vi "IMAQ FPGA Image Transfer to Target U64.vi"(7 "Write Timeout (ms)":i32=5000, 8 "error in (no error)":errorcluster, 9 "DMA FIFO Reference In":refnum<k20>, 10 "Maximum Pixels per Write":i32=-1, 11 "Image":T1) -> (0 "error out":errorcluster, 1 "DMA FIFO Reference Out":refnum<k20>, 3 "Image Out":T1)   [LabVIEW 2017, in "NI_VDM_FPGA_Basics.lvlib"]
doc: "Transfers an image from the host processor to the target FPGA via a DMA FIFO."
uses:
  <vilib>/visionFPGA/NI_VDM_FPGA_Basics.lvlib
  <vilib>/vision/Image Controls.llb/IMAQ Image.ctl
  <vilib>/rvi/errors/niLvFpgaAdjustHostInterfaceError.vi
  <vilib>/rvi/interface/nirviMethod/nirviMethod.xnode
  <vilib>/rvi/errors/niLvFpgaMergeErrorWithErrorCode.vi
  <vilib>/FPGAPlugInAG/Dynamic/niLvFpga_WriteFifo_Dynamic.vi
  <vilib>/FPGAPlugInAG/Dynamic/niLvFpga_AcquireWriteRegionFifo_Dynamic.vi
  <vilib>/vision/EDVR.llb/IMAQ ImageToEDVR 2D U64.vi
  nivissvc.dll
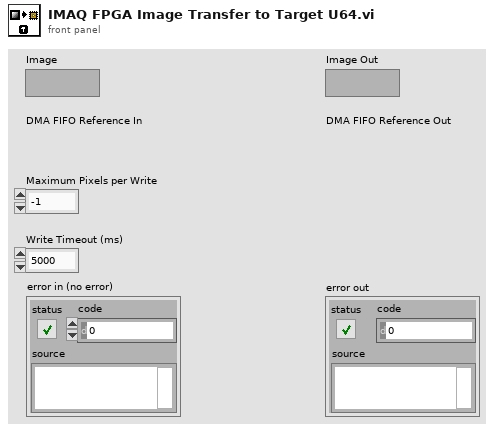
[diagram p1: front panel]
types:
  T1 = typedef "IMAQ Image.ctl" = refnum<image>
  T2 = typedef "Image Type" = u32
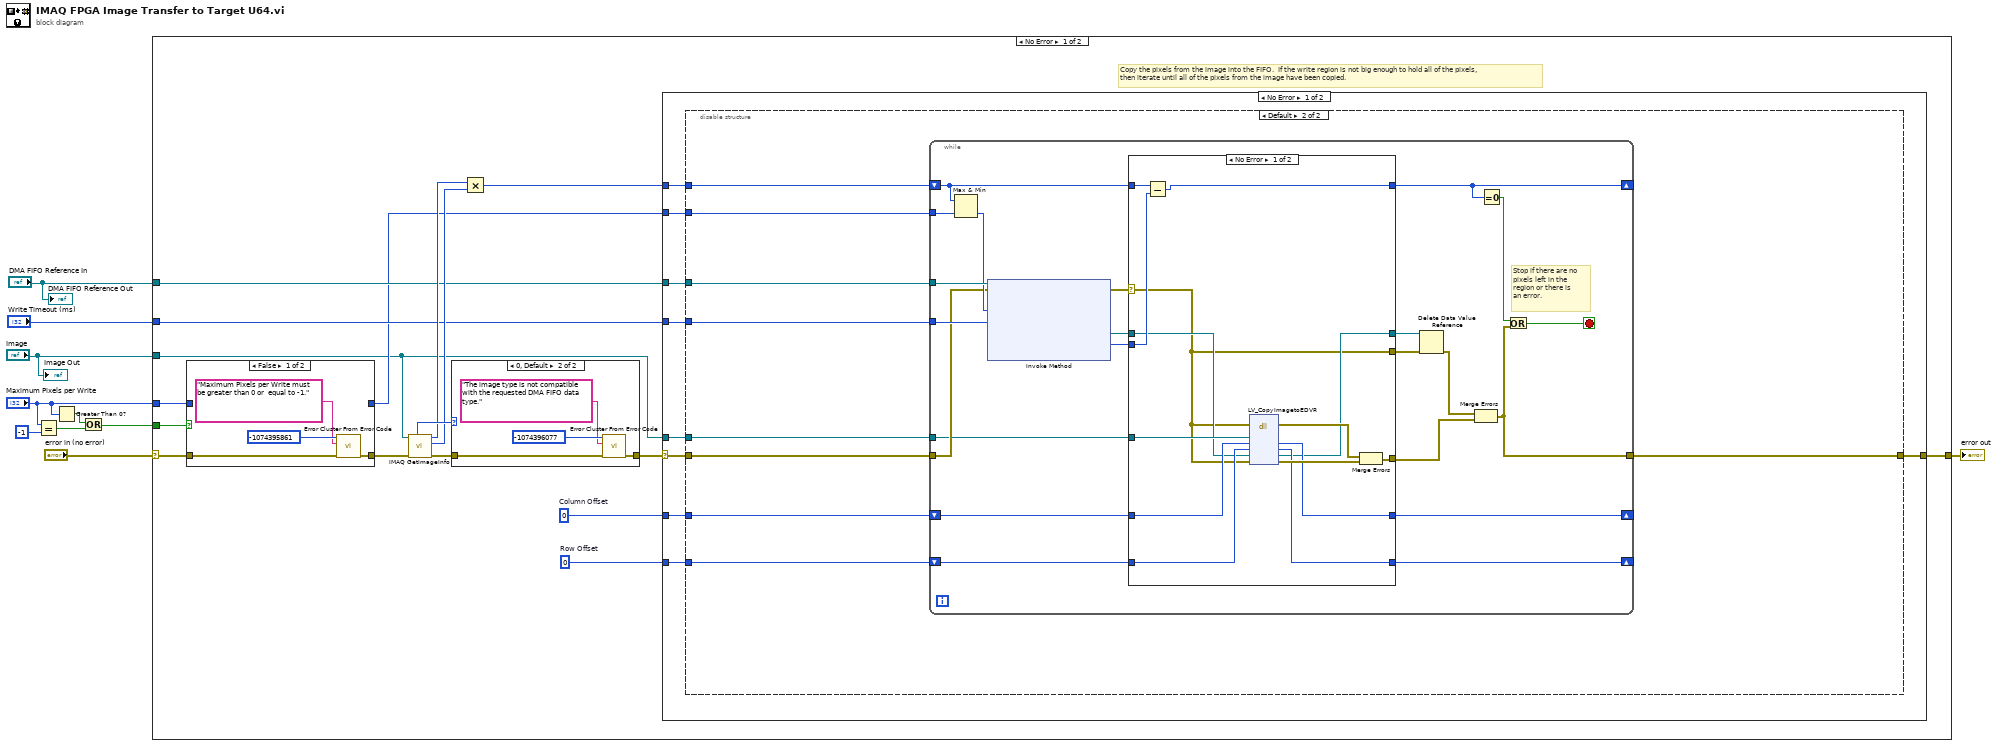
[diagram p0: block diagram]
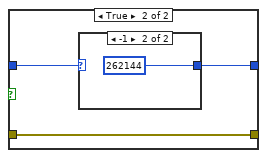
[diagram p2: hidden frame]
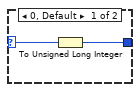
[diagram p3: hidden frame]
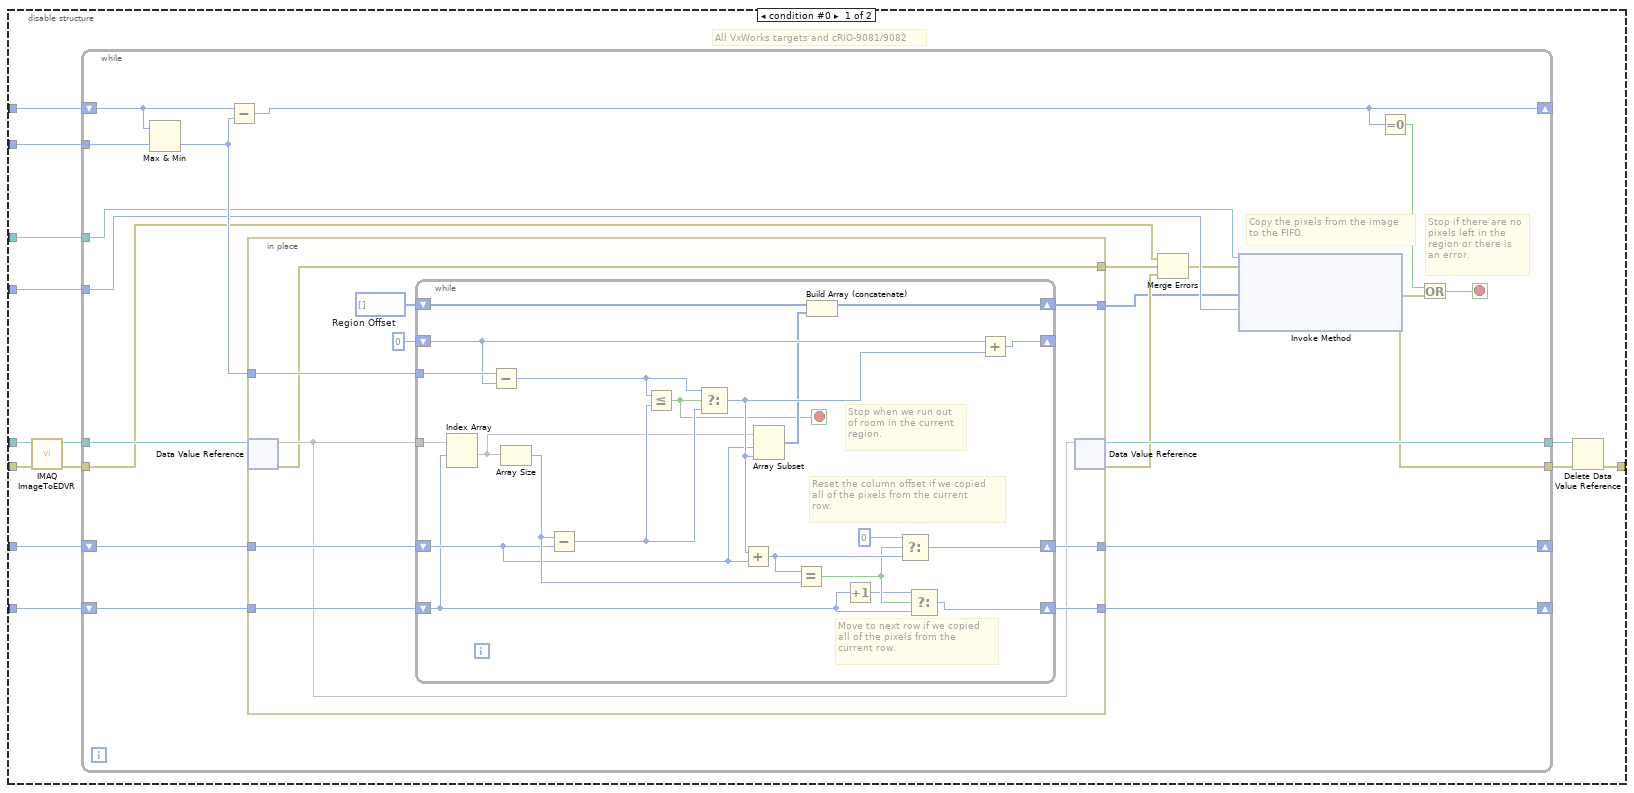
[diagram p4: hidden frame]
diagram:
  n1 = Equal?(x="Maximum Pixels per Write", y=-1) -> (x = y?=w6:bool)
  n2 = Greater Than 0?(x="Maximum Pixels per Write") -> (x > 0?=w7:bool)
  n3 = Or(x=w7, y=w6) -> (x .or. y?=w5:bool)
  n4 = case shown="No Error" "error in (no error)" {
    selector: "error in (no error)" -> [w11 w167]
    tunnel: "DMA FIFO Reference In" -> [w22 _]
    tunnel: "Write Timeout (ms)" -> [w21 _]
    tunnel: w5 -> [w18 _]
    tunnel: "Maximum Pixels per Write" -> [w15 _]
    tunnel: "Image" -> [w13 _]
    tunnel: [w12 w167] -> w2
    frame No Error {
      w19 = u32 0  # Row Offset
      w20 = u32 0  # Column Offset
      # "Copy the pixels from the image into the FIFO.  If the write region is not big enough to hold all of the pixels,\nthen iterate until all of the pixels from the image have been copied."
      n5 = case shown="False" w18 {
        tunnel: w11 -> [w29 w34]
        tunnel: [w28 w34] -> w17
        tunnel: w15 -> [_ w33]
        tunnel: [_ w32] -> w16
        frame False {
          n6 = call <vilib>:"Error Cluster From Error Code.vi"("error in (no error)"=w29, "error message (\"\")"="Maximum Pixels per Write must be greater than 0 or  equal to -1." ("error message (\"\")"), "error code (0)"=-1074395861) -> ("error out"=w28:errorcluster)  [unwired: 6 in]
        }
        frame True {
          n7 = case shown="-1" w33 {
            selector: w33 -> [w36 _]
            tunnel: [w35 u32 262144 ("Maximum Pixels per Write")] -> w32
            frame 0, Default {
              n8 = To Unsigned Long Integer(number=w36) -> (unsigned 32bit integer=w35:u32)
            }
            frame -1 {
            }
          }
        }
      }
      n9 = call "IMAQ GetImageInfo"("error in (no error)"=w17, "Image"=w13) -> ("error out"=w26:errorcluster, "Y Resolution"=w24:i32, "X Resolution"=w25:i32, "Image Type"=w27:T2)  [unwired: 2 in, 4 out]
      n10 = case shown="0, Default" w27 {
        tunnel: w26 -> [w162 w164]
        tunnel: [w162 w163] -> w14
        frame 6 {
          # "Allowed types are:\nRGB (U64)"
        }
        frame 0, Default {
          n11 = call <vilib>:"Error Cluster From Error Code.vi"("error in (no error)"=w164, "error message (\"\")"="The image type is not compatible with the requested DMA FIFO data type." ("error message (\"\")"), "error code (0)"=-1074396077) -> ("error out"=w163:errorcluster)  [unwired: 6 in]
        }
      }
      n12 = Multiply(x=w25, y=w24) -> (x*y=w23:i32)
      n13 = case shown="No Error" w14 {
        selector: w14 -> [w44 w161]
        tunnel: w23 -> [w39 _]
        tunnel: w20 -> [w45 _]
        tunnel: w19 -> [w46 _]
        tunnel: w22 -> [w41 _]
        tunnel: [w38 w161] -> w12
        tunnel: w16 -> [w40 _]
        tunnel: w21 -> [w42 _]
        tunnel: w13 -> [w43 _]
        frame No Error {
          n14 = disable-structure shown="Default" {
            disable-tunnel: w39 -> [w59 w119]
            disable-tunnel: w45 -> [w58 w118]
            disable-tunnel: w46 -> [w57 w117]
            disable-tunnel: w41 -> [w56 w116]
            disable-tunnel: [w47 w115] -> w38
            disable-tunnel: w40 -> [w55 w114]
            disable-tunnel: w42 -> [w54 w113]
            disable-tunnel: w44 -> [w52 w112]
            disable-tunnel: w43 -> [w53 w111]
            frame condition #0 {
              # "All VxWorks targets and cRIO-9081/9082"
              n15 = call-poly <vilib>:"IMAQ ImageToEDVR.vi"("error in (no error)"=w52, "Image"=w53) -> ("error out"=w50:errorcluster, "EDVR 2D U64"=w51:refnum<data-value>)  [unwired: 7 in, 1 out]
              n16 = while {
                shift-right: [w73] -> _
                shift-left: w59 -> [w70]
                tunnel: w51 -> [w79]
                shift-right: [w75] -> _
                shift-left: w58 -> [w77]
                shift-right: [w78] -> _
                shift-left: w57 -> [w76]
                tunnel: w56 -> [w64]
                tunnel: [w74] -> w49
                tunnel: [w62] -> w48
                tunnel: w55 -> [w69]
                tunnel: w54 -> [w65]
                tunnel: w50 -> [w60]
                stop <- w72 stop-if-true
                # "Copy the pixels from the image\nto the FIFO."
                # "Stop if there are no\npixels left in the \nregion or there is\nan error."
                n17 = Max & Min(x=w70, y=w69) -> (min(x,y)=w68:u32)  [unwired: 1 out]
                n18 = Subtract(x=w70, y=w68) -> (x-y=w73:u32)
                n19 = in-place {
                  in-place-border: w68 -> [w87]
                  in-place-border: [w89] -> w78
                  in-place-border: w77 -> [w86]
                  in-place-border: w76 -> [w84]
                  in-place-border: [w85] -> w75
                  in-place-border: [w81] -> w67
                  in-place-border: [w80] -> w61
                  w88 = u32 0  # Region Offset
                  n20 = in-place-dvr #1(w79) -> (w83:u64[][], w81:errorcluster)
                  n21 = while {
                    tunnel: w83 -> [w96]
                    shift-right: [w108] -> _
                    shift-left: w88 -> [w107]
                    tunnel: w87 -> [w110]
                    shift-right: [w101] -> w85
                    shift-left: w86 -> [w97]
                    shift-right: [w91] -> w80
                    shift-left: u8[] [] -> [w93]
                    shift-right: [w98] -> w89
                    shift-left: w84 -> [w94]
                    stop <- w90 stop-if-true
                    # "Stop when we run out\nof room in the current\nregion."
                    # "Reset the column offset if we copied\nall of the pixels from the current\nrow."
                    # "Move to next row if we copied\nall of the pixels from the\ncurrent row."
                    n22 = Index Array(array=w96, index (row)=w94) -> (element=w95:u64[])  [unwired: 1 in]
                    n23 = Subtract(x=w110, y=w107) -> (x-y=w109:u32)
                    n24 = Array Size(array=w95) -> (size(s)=w106:i32)
                    n25 = Subtract(x=w106, y=w97) -> (x-y=w104:u32)
                    n26 = Less Or Equal?(x=w109, y=w104) -> (x <= y?=w90:bool)
                    n27 = Select(t=w109, s=w90, f=w104) -> (s? t:f=w105:u32)
                    n28 = Add(x=w105, y=w97) -> (x+y=w102:u32)
                    n29 = Array Subset(array=w95, index=w97, length=w105) -> (w92:u64[])
                    n30 = Equal?(x=w102, y=w106) -> (x = y?=w100:bool)
                    n31 = Build Array (concatenate)(w93, w92) -> (w91:u64[])
                    n32 = Increment(x=w94) -> (x+1=w99:u32)
                    n33 = Select(t=u32 0 ("Elements In Region"), s=w100, f=w102) -> (s? t:f=w101:u32)
                    n34 = Select(t=w99, s=w100, f=w94) -> (s? t:f=w98:u32)
                    n35 = Add(x=w107, y=w105) -> (x+y=w108:u32)
                  }
                  n36 = in-place-dvr #1(w83) -> (w74:refnum<data-value>, w66:errorcluster)
                }
                n37 = Merge Errors(w60, w67, w66) -> (w63:errorcluster)
                n38 = xnode "Invoke Method"("FPGA VI Reference In"=w64, "error in"=w63, "Data"=w61, "Timeout (ms)"=w65) -> ("error out"=w62:errorcluster)  [unwired: 2 out]
                n39 = Equal To 0?(x=w73) -> (x = 0?=w71:bool)
                n40 = Or(x=w71, y=w62) -> (x .or. y?=w72:bool)
              }
              n41 = Delete Data Value Reference(data value reference=w49, error in=w48) -> (error out=w47:errorcluster)  [unwired: 1 out]
            }
            frame condition #1 (active) {
              n42 = while {
                shift-right: [w129] -> _
                shift-left: w119 -> [w124]
                shift-right: [w136] -> _
                shift-left: w118 -> [w138]
                shift-right: [w139] -> _
                shift-left: w117 -> [w137]
                tunnel: w116 -> [w135]
                tunnel: [w127] -> w115
                tunnel: w114 -> [w123]
                tunnel: w113 -> [w122]
                tunnel: w112 -> [w121]
                tunnel: w111 -> [w120]
                stop <- w128 stop-if-true
                # "Stop if there are no\npixels left in the \nregion or there is\nan error."
                n43 = Max & Min(x=w124, y=w123) -> (min(x,y)=w125:u32)  [unwired: 1 out]
                n44 = xnode "Invoke Method"("FPGA VI Reference In"=w135, "error in"=w121, "Number of Elements"=w125, "Timeout (ms)"=w122) -> ("error out"=w134:errorcluster, "Write Region Reference"=w141:refnum<data-value>, "Elements In Region"=w140:u32)  [unwired: 2 out]
                n45 = case shown="No Error" w134 {
                  selector: w134 -> [w142 w157]
                  tunnel: w124 -> [w155 w160]
                  tunnel: [w154 w160] -> w129
                  tunnel: w141 -> [w148 w156]
                  tunnel: w140 -> [w153 _]
                  tunnel: [w144 w158] -> w139
                  tunnel: w138 -> [w151 w159]
                  tunnel: w137 -> [w150 w158]
                  tunnel: [w145 w159] -> w136
                  tunnel: [w143 w156] -> w133
                  tunnel: [w142 w157] -> w132
                  tunnel: [w146 _] -> w130
                  tunnel: w120 -> [w152 _]
                  frame No Error {
                    n46 = Subtract(x=w155, y=w153) -> (x-y=w154:u32)
                    n47 = dll-call lib="nivissvc.*" fn="LV_CopyImagetoEDVR" label="LV_CopyImageToEDVR"(error in=w142, "image"=w152, "xImageOffset"=w151, "yImageOffset"=w150, "EDVR"=w148, "error"=w142) -> (error out=w149:errorcluster, "xImageOffset"=w145:u32, "yImageOffset"=w144:u32, "EDVR"=w143:refnum<data-value>, "error"=w147:errorcluster)  [unwired: 4 in, 1 out]
                    n48 = Merge Errors(w149, w147) -> (w146:errorcluster)
                  }
                  frame Error {
                  }
                }
                n49 = Delete Data Value Reference(data value reference=w133, error in=w132) -> (error out=w131:errorcluster)  [unwired: 1 out]
                n50 = Merge Errors(w131, w130) -> (w127:errorcluster)
                n51 = Equal To 0?(x=w129) -> (x = 0?=w126:bool)
                n52 = Or(x=w126, y=w127) -> (x .or. y?=w128:bool)
              }
            }
          }
        }
        frame Error {
        }
      }
    }
    frame Error {
    }
  }
  "error out" <- w2
  "Image Out" <- "Image"
  "DMA FIFO Reference Out" <- "DMA FIFO Reference In"
